vi "SHIMSsub.vi"(10 "Numeric":i16, 11 "VISA Refnum in":refnum<visa-resource-name>) -> ()   [LabVIEW 2019]
uses:
  <vilib>/Instr/_visa.llb/VISA Configure Serial Port (Instr).vi
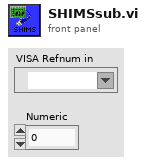
[diagram p1: front panel]
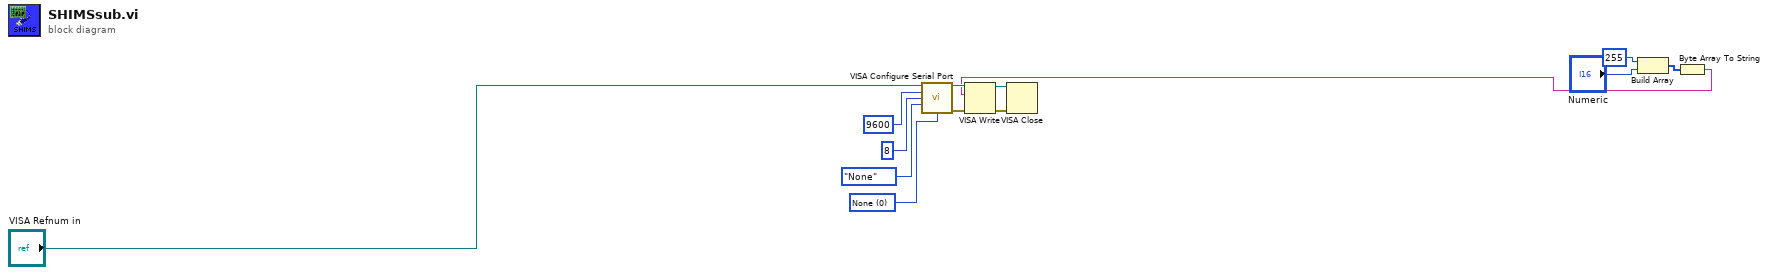
[diagram p0: block diagram]
diagram:
  w7 = u16 0 items=["None", "XON/XOFF", "RTS/CTS", "XON/XOFF & RTS/CTS", "DTR/DSR", "XON/XOFF & DTR/DSR"] ("flow control (0:none)")
  n1 = call-poly "VISA Configure Serial Port"("VISA resource name"="VISA Refnum in", "baud rate (9600)"=u32 9600, "data bits (8)"=u16 8, "parity (0:none)"=enum16{"None", "Odd", "Even", "Mark", "Space"}."None", "flow control (0:none)"=w7) -> ("VISA resource name out"=w13:refnum<visa-resource-name>, "error out"=w10:errorcluster)  [unwired: 1 in, 8 out]
  n2 = Build Array(i16 255 ("element"), "Numeric") -> (w2:i16[])
  n3 = Byte Array To String(unsigned byte array=w2) -> (string=w12:string)
  n4 = VISA Write(VISA resource name=w13, write buffer=w12, error in (no error)=w10) -> (VISA resource name out=w9:refnum<visa-resource-name>, error out=w8:errorcluster)  [unwired: 1 out]
  n5 = VISA Close(VISA resource name=w9, error in (no error)=w8) -> ()  [unwired: 1 out]
